vi "set and reset slider tabs.vi"(11 "Set(T)/Reset(F)":bool) -> ()   [LabVIEW 2012]
uses:
  <vilib>/Utility/miscctls.llb/LVPositionTypeDef.ctl
  <vilib>/Utility/miscctls.llb/LVBoundsTypeDef.ctl
  GFG/GFGfpRefGet.vi
  GFG/GFG library.lvlib
panel:
  out "String":string
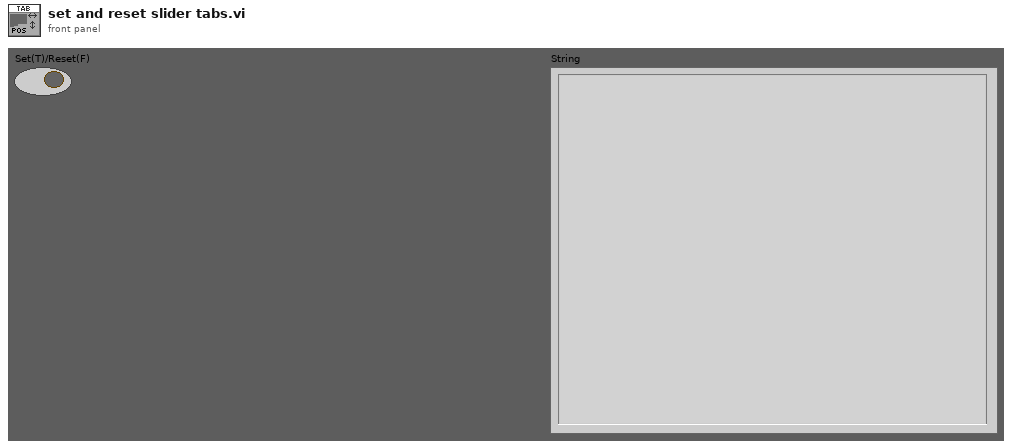
[diagram p1: front panel]
types:
  T1 = typedef "LVPositionTypeDef.ctl" = cluster{"Left":i32, "Top":i32}
  T2 = typedef "LVBoundsTypeDef.ctl" = cluster{"Width":u32, "Height":u32}
  T3 = cluster{"WaveformChartRef":refnum<vi>, "DigitalRef":refnum<vi>, "ArrayRef":refnum<vi>, "TabControlRef":refnum<vi>, "EnumRef":refnum<vi>, "RingRef":refnum<vi>, "BooleanRef":refnum<vi>, "KnobRef":refnum<vi>, "SlideRef":refnum<vi>, "PathRef":refnum<vi>, "StringRef":refnum<vi>, "ComboBox":refnum<vi>, "WaveformGraphRef":refnum<vi>}
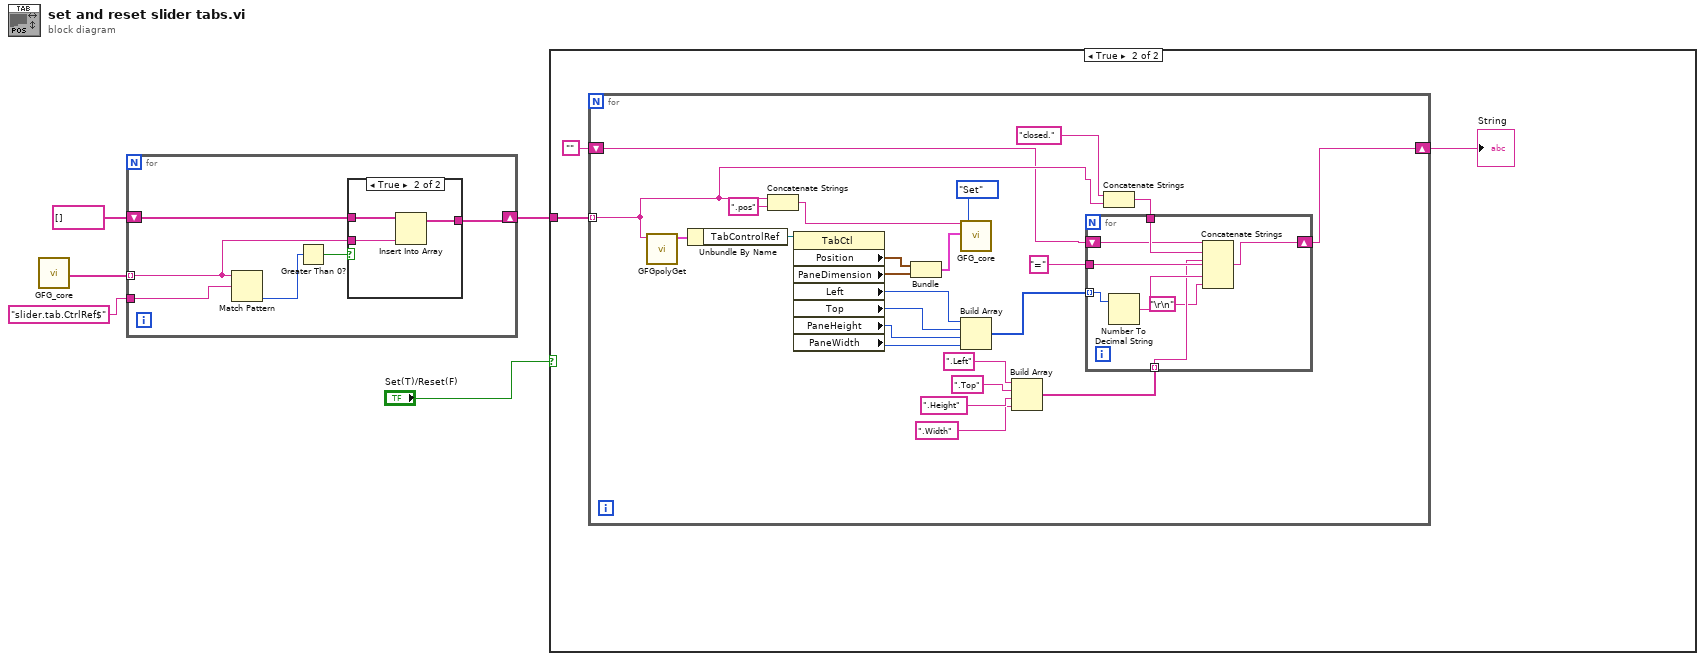
[diagram p0: block diagram]
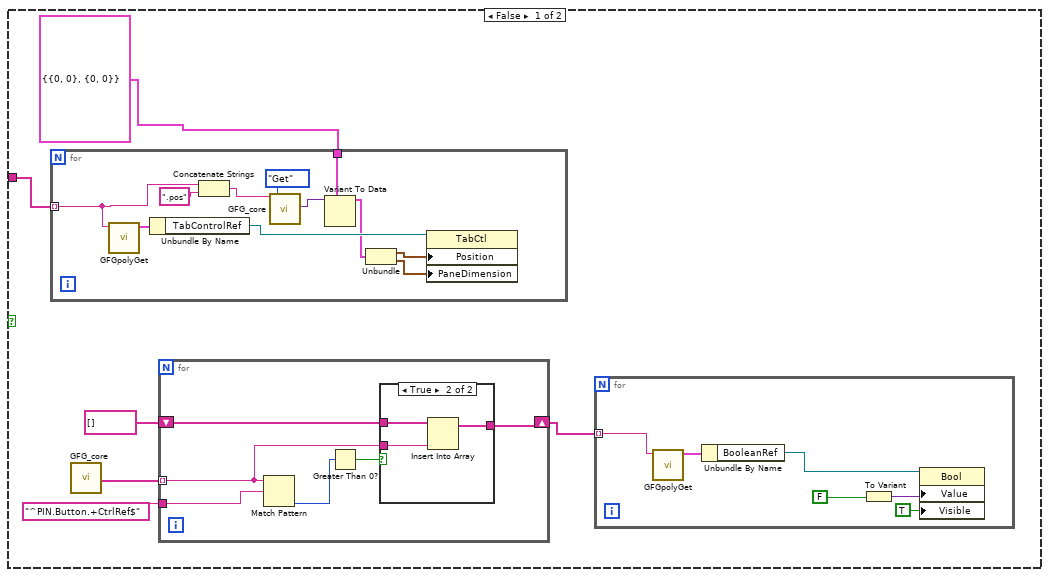
[diagram p2: hidden frame]
diagram:
  n1 = call "GFG_core.vi"() -> ("All Variable Names Out"=w5:string[])  [unwired: 13 in, 6 out]
  n2 = for {
    tunnel: w5 -> [w6] mode=indexing
    shift-right: [w9] -> w2
    shift-left: string[] [] ("All Variable Names Out") -> [w10]
    tunnel: "slider.tab.CtrlRef$" ("regular expression") -> [w7]
    n3 = Match Pattern(string=w6, regular expression=w7) -> (offset past match=w11:i32)  [unwired: 1 in, 3 out]
    n4 = Greater Than 0?(x=w11) -> (x > 0?=w8:bool)
    n5 = case shown="True" w8 {
      tunnel: w10 -> [w12 w15]
      tunnel: [w12 w14] -> w9
      tunnel: w6 -> [_ w13]
      frame False {
      }
      frame True {
        n6 = Insert Into Array(array=w15, new element=w13) -> (w14:string[])  [unwired: 1 in]
      }
    }
  }
  n7 = case shown="True" "Set(T)/Reset(F)" {
    tunnel: w2 -> [w21 w51]
    frame False {
      n8 = for {
        tunnel: w21 -> [w44] mode=indexing
        tunnel: cluster{"Position":T1, "PaneDimension":T2} {"Position"={"Left"=0, "Top"=0}, "PaneDimension"={"Width"=0, "Height"=0}} ("output cluster") -> [w42]
        n9 = call-poly "GFGpolyGet.vi"("Variable Name in"=w44) -> ("output cluster"=w47:T3)  [unwired: 9 in, 1 out]
        n10 = Unbundle By Name(w47) -> ("TabControlRef"=w46:refnum<vi>)
        n11 = Concatenate Strings(w44, ".pos" ("string")) -> (w41:string)
        n12 = call "GFG_core.vi"("Variable Name in"=w41, "Action"=enum16{"Init", "Set", "Get"}."Get") -> ("Variant Out"=w43:variant)  [unwired: 11 in, 6 out]
        n13 = Variant To Data(type=w42, Variant=w43) -> (data=w40:cluster{"Position":T1, "PaneDimension":T2})  [unwired: 1 in, 1 out]
        n14 = Unbundle(w40) -> ("Position"=w39:T1, "PaneDimension"=w38:T2)
        n15 = property class="TabCtl"(reference=w46, "Position"=w39, "PaneDimension"=w38) -> ()  [unwired: 1 in, 2 out]
      }
      n16 = call "GFG_core.vi"() -> ("All Variable Names Out"=w18:string[])  [unwired: 13 in, 6 out]
      n17 = for {
        tunnel: w18 -> [w28] mode=indexing
        shift-right: [w31] -> w17
        shift-left: string[] [] ("All Variable Names Out") -> [w32]
        tunnel: "^PIN.Button.+CtrlRef$" ("regular expression") -> [w29]
        n18 = Match Pattern(string=w28, regular expression=w29) -> (offset past match=w33:i32)  [unwired: 1 in, 3 out]
        n19 = Greater Than 0?(x=w33) -> (x > 0?=w30:bool)
        n20 = case shown="True" w30 {
          tunnel: w32 -> [w34 w37]
          tunnel: [w34 w36] -> w31
          tunnel: w28 -> [_ w35]
          frame False {
          }
          frame True {
            n21 = Insert Into Array(array=w37, new element=w35) -> (w36:string[])  [unwired: 1 in]
          }
        }
      }
      n22 = for {
        tunnel: w17 -> [w25] mode=indexing
        n23 = call-poly "GFGpolyGet.vi"("Variable Name in"=w25) -> ("output cluster"=w27:T3)  [unwired: 9 in, 1 out]
        n24 = Unbundle By Name(w27) -> ("BooleanRef"=w26:refnum<vi>)
        n25 = To Variant(anything=FALSE ("Set(T)/Reset(F)")) -> (Variant=w24:variant)
        n26 = property class="Bool"(reference=w26, "Value"=w24, "Visible"=TRUE) -> ()  [unwired: 1 in, 2 out]
      }
    }
    frame True {
      n27 = for {
        tunnel: w51 -> [w66] mode=indexing
        shift-right: [w52] -> w49
        shift-left: "" -> [w53]
        n28 = call-poly "GFGpolyGet.vi"("Variable Name in"=w66) -> ("output cluster"=w74:T3)  [unwired: 9 in, 1 out]
        n29 = Unbundle By Name(w74) -> ("TabControlRef"=w73:refnum<vi>)
        n30 = Concatenate Strings(w66, ".pos" ("string")) -> (w71:string)
        n31 = property class="TabCtl"(reference=w73) -> ("Position"=w69:T1, "PaneDimension"=w70:T2, "Left"=w63:i32, "Top"=w62:i32, "PaneHeight"=w61:u32, "PaneWidth"=w60:u32)  [unwired: 1 in, 2 out]
        n32 = Bundle("Position"=w69, "PaneDimension"=w70) -> (w68:cluster{"Position":T1, "PaneDimension":T2})  [unwired: 1 in]
        n33 = call "GFG_core.vi"("Variable Name in"=w71, "Variant in"=w68, "Action"=enum16{"Init", "Set", "Get"}."Set") -> ()  [unwired: 10 in, 7 out]
        n34 = Build Array(w63, w62, w61, w60) -> (w55:u32[])
        n35 = Build Array(".Left" ("string"), ".Top" ("string"), ".Height" ("string"), ".Width" ("string")) -> (w54:string[])
        n36 = Concatenate Strings("closed." ("string"), w66) -> (w64:string)
        n37 = for {
          tunnel: "=" ("string") -> [w83]
          tunnel: w64 -> [w82]
          tunnel: w55 -> [w80] mode=indexing
          tunnel: w54 -> [w79] mode=indexing
          shift-right: [w76] -> w52
          shift-left: w53 -> [w77]
          n38 = Number To Decimal String(number=w80) -> (decimal integer string=w81:string)  [unwired: 1 in]
          n39 = Concatenate Strings(w77, w82, w79, w83, w81, "\r\n") -> (w76:string)
        }
      }
      "String" <- w49
    }
  }
